vi "Put file.vi"(8 "error in (no error)":errorcluster, 9 "Local path":path, 10 "Remote path":string, 11 "FTP in":refnum<class "FTP.lvclass">) -> (0 "error out":errorcluster, 3 "FTP out":refnum<class "FTP.lvclass">)   [LabVIEW 2015, in "RT Management.lvlib" / "FTP.lvclass"]
uses:
  FTP.lvclass
  FTP.lvclass/FTP.ctl
  File Transfer Behavior/Fix path [scalar].vi
  Get Session.vi
  <vilib>/Utility/error.llb/Trim Whitespace.vi
  File Transfer Behavior/File Transfer Behavior.lvclass
  <vilib>/FTP/NI_FTP.lvlib
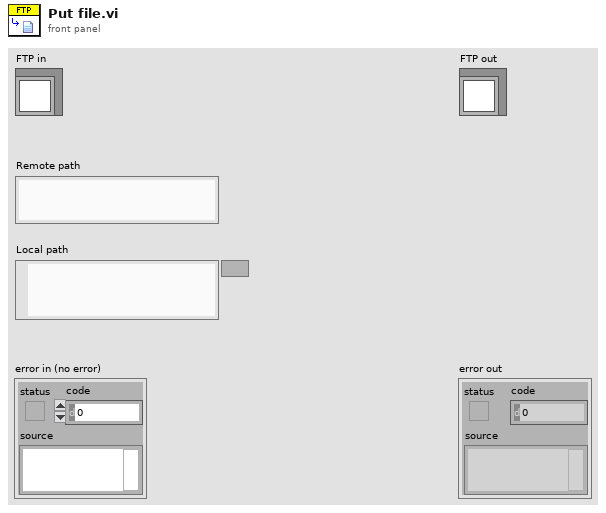
[diagram p1: front panel]
types:
  T1 = cluster{"remote path":string, "local path":path, "binary":bool, "data":string}
  T2 = typedef "NI_FTP.lvlib/FTP Session.ctl" = refnum<k5>
  T3 = cluster{"remote path":string, "local path":path, "binary":bool, "data":string}[]
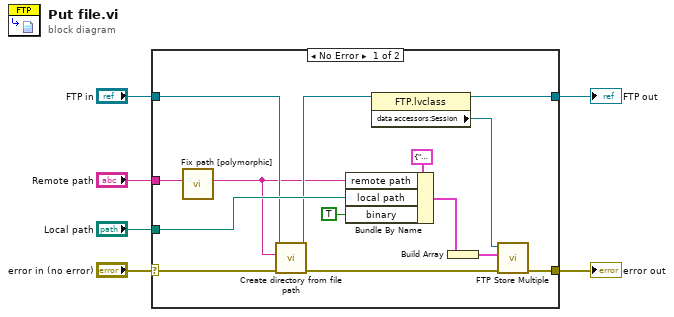
[diagram p0: block diagram]
diagram:
  n1 = case shown="No Error" "error in (no error)" {
    selector: "error in (no error)" -> [w13 w22]
    tunnel: [w20 w22] -> w5
    tunnel: "Remote path" -> [w9 _]
    tunnel: "Local path" -> [w19 _]
    tunnel: "FTP in" -> [w12 w21]
    tunnel: [w7 w21] -> w2
    frame No Error {
      n2 = call-poly "Fix path [polymorphic].vi"("Path in"=w9) -> ("Path out"=w8:string)  [unwired: 8 in, 2 out]
      n3 = call "Create directory from file path.vi"("error in (no error)"=w13, "File path"=w8, "File Transfer Behavior in"=w12) -> ("error out"=w10:errorcluster, "File Transfer Behavior out"=w11:refnum<class "FTP.lvclass">)  [unwired: 7 in]
      n4 = Bundle By Name(cluster=T1 {"remote path"="", "local path"=path "", "binary"=FALSE, "data"=""} ("transfer spec"), "remote path"=w8, "local path"=w19, "binary"=TRUE ("active (T)")) -> (w16:T1)
      n5 = property class="FTP.lvclass"(reference=w11) -> (reference out=w7:refnum<class "FTP.lvclass">, "data accessors:Session"=w18:T2)  [unwired: 1 in, 1 out]
      n6 = Build Array(w16) -> (w15:T3)
      n7 = call <vilib>:"FTP Store Multiple.vi"("error in (no error)"=w10, "file specifications"=w15, "ftp session"=w18) -> ("error out"=w20:errorcluster)  [unwired: 1 in, 7 out]
    }
    frame Error {
    }
  }
  "error out" <- w5
  "FTP out" <- w2
